vi "Init Msg.vi"(10 "Msg Input":refnum<class "Msg Input.lvclass">) -> (3 "Start Msg out":refnum<class "Start Msg.lvclass">)   [LabVIEW 2020, in "jettl.lvlib" / "Start jettl Msg.lvlib" / "Start Msg.lvlib" / "Start Msg.lvclass"]
doc: "jettl 6.14.1.98\nNathan Davis - Nathan Davis\nCopyright (c) 2026, Nathan Davis\nMIT"
uses:
  Start Msg.lvclass
  Msg Input/Msg Input.lvclass
  Start Msg.lvclass/Start Msg.ctl
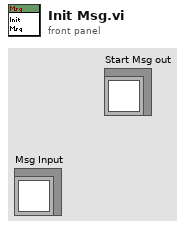
[diagram p1: front panel]
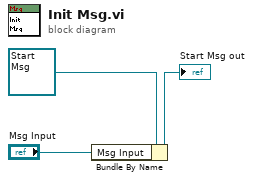
[diagram p0: block diagram]
diagram:
  n1 = Bundle By Name(cluster=refnum<class "Start Msg.lvclass"> refnum ("TEMPLATE Msg out"), "Msg Input"="Msg Input") -> (→"Start Msg out":refnum<class "Start Msg.lvclass">)
